vi "Parse.vi"(8 "Error In":errorcluster, 11 "object in":refnum<class "2021_3.lvclass">) -> (0 "Error Out":errorcluster, 3 "object out":refnum<class "2021_3.lvclass">)   [LabVIEW 2020, in "2021_3.lvclass"]
uses:
  2021_3.lvclass
  2021_3.lvclass/2021_3.ctl
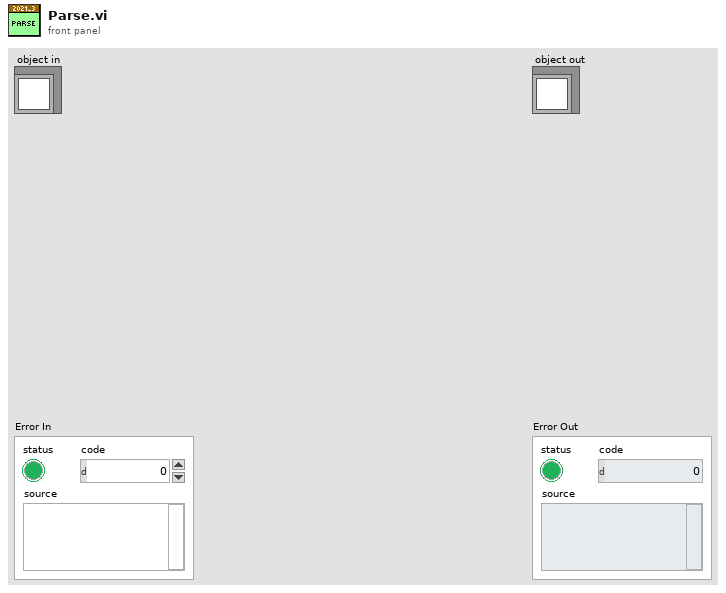
[diagram p1: front panel]
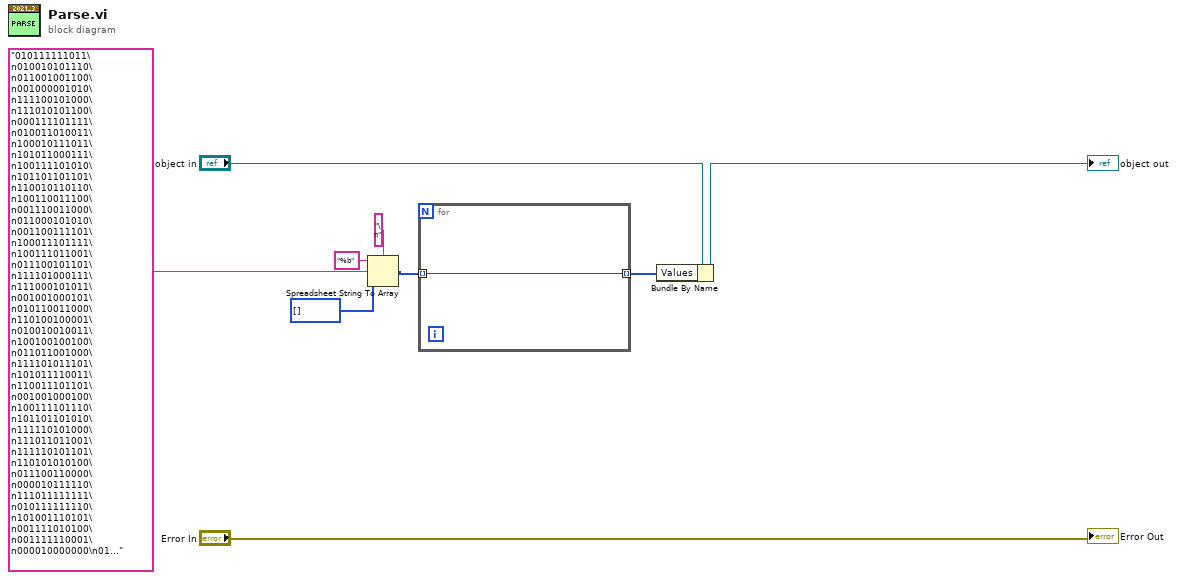
[diagram p0: block diagram]
diagram:
  n1 = Spreadsheet String To Array(delimiter (Tab)="\n", format string="%b", spreadsheet string="010111111011\n010010101110\n011001001100\n001000001010\n111100101000\n111010101100\n000111101111\n010011010011\n100010111011\n101011000111\n100111101010\n101101101101\n110010110110\n100110011100\n001110011000\n011000101010\n001100111101\n100011101111\n100111011001\n011100101101\n111101000111\n111000101011\n001001000101\n010110011000\n110100100001\n010010010011\n100100100100\n011011001000\n111101011101\n101011110011\n110011101101\n001001000100\n100111101110\n101101101010\n111110101000\n111011011001\n111110101101\n110101010100\n011100110000\n000010111110\n111011111111\n010111111110\n101001110101\n001111010100\n001111110001\n000010000000\n01..." ("PuzzleInput"), array type (2D Dbl)=u32[] []) -> (array=w3:u32[])
  n2 = for {
    tunnel: w3 -> [w10] mode=indexing
    tunnel: [w10] -> w1 mode=indexing
  }
  n3 = Bundle By Name(cluster="object in", "Values"=w1) -> (→"object out":refnum<class "2021_3.lvclass">)
  "Error Out" <- "Error In"
